vi "KalmanMain.vi"() -> ()   [LabVIEW 2017]
uses:
  <vilib>/Analysis/Matrix/Datatypes/RealMatrix.ctl
  4782e2db-7f08-4414-a468-fee53f76426c.vi
  <vilib>/Analysis/baseanly.llb/Real A x B.vi
  <vilib>/Analysis/Matrix/Numeric/Add/Add - RM,RM.vi
  <vilib>/Analysis/7linalg.llb/Create Special Real Matrix.vi
  <vilib>/Analysis/baseanly.llb/Real Inverse Matrix.vi
  <vilib>/Analysis/Matrix/Numeric/Subtract/Subtract - RM,RM.vi
  <vilib>/Analysis/NI_AALBase.lvlib
  <vilib>/Analysis/Matrix/NI_Matrix.lvlib
  <vilib>/Analysis/NI_AALPro.lvlib
panel:
  in  "delay":u32=500
  out "P 2":T1
  out "Xhat 2":T1
  in  "Xhat":T1=[[0.0], [0.0]]
  in  "Q":T1=[[1.0, 0.0], [0.0, 1.0]]
  in  "R":T1=[[1.0]]
  in  "H":T1=[[1.0, 0.0]]
  in  "A":T1=[[1.0, 1.0], [0.0, 1.0]]
  in  "P":T1=[[10.0, 0.0], [0.0, 10.0]]
  in  "Measurements":dbl[](array[numeric])=[1.0, 2.0, 3.0, 4.0]
  out "XY Graph":T2(graph)
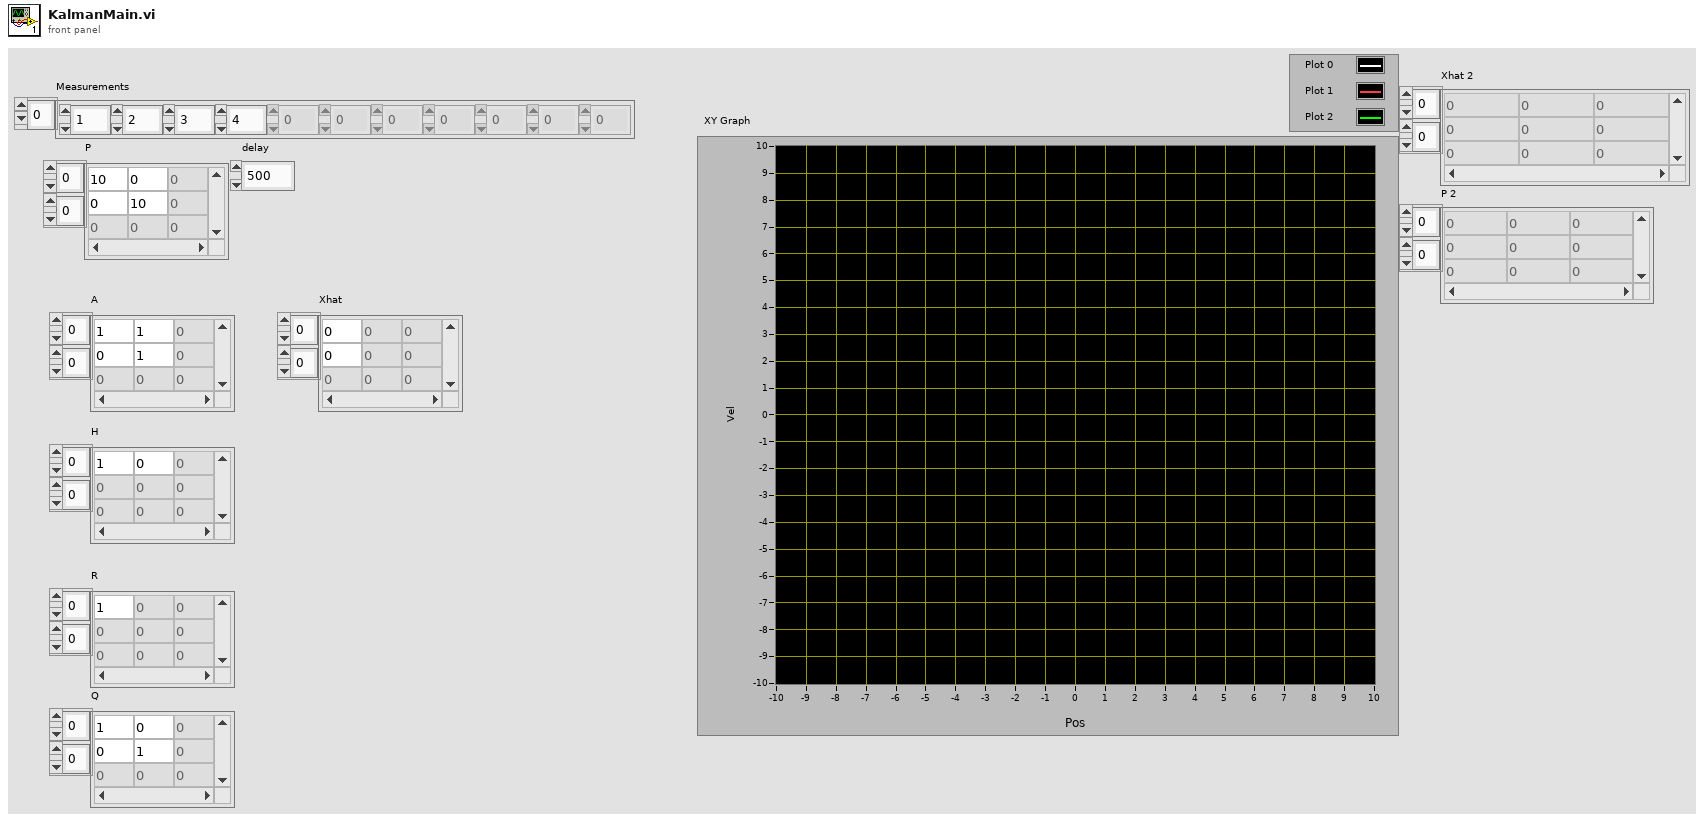
[diagram p1: front panel]
types:
  T1 = typedef "NI_Matrix.lvlib/RealMatrix.ctl" = dbl[][]
  T2 = cluster{"A x Vector":dbl[], "A x Vector":dbl[]}[]
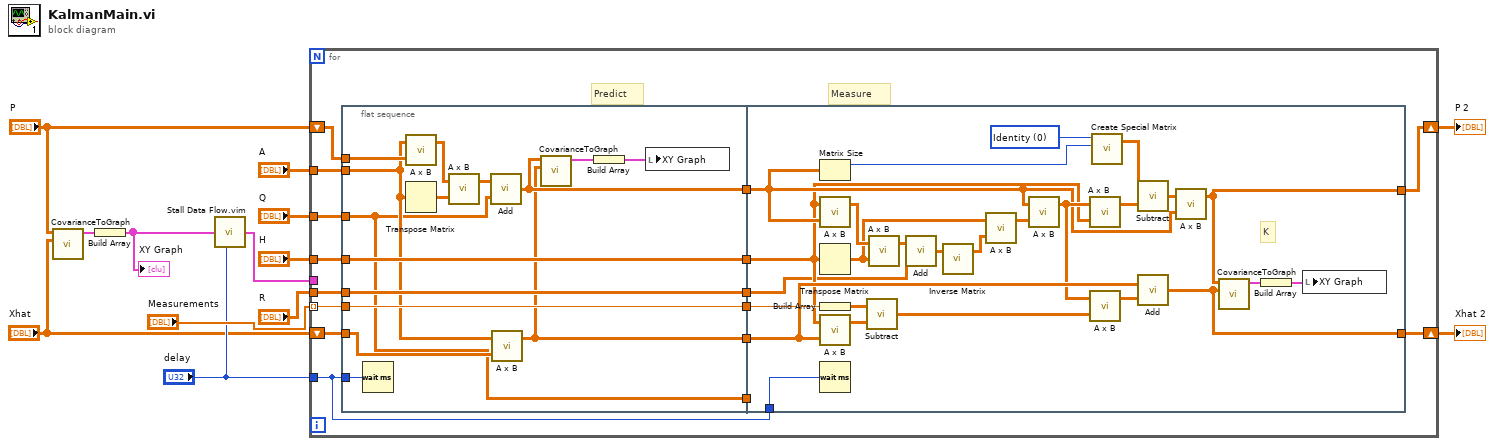
[diagram p0: block diagram]
diagram:
  n1 = call "CovarianceToGraph.vi"("Mu"="Xhat", "covariance matrix"="P") -> ("XY Graph"=w13:cluster{cdb[], cdb[]})  [unwired: 9 in]
  n2 = Build Array(w13) -> (w4:cluster{cdb[], cdb[]}[])
  "XY Graph" <- w4
  n3 = call "Stall Data Flow.vim"("value in"=w4, "milliseconds to wait"="delay") -> ("value out"=w3:cluster{cdb[], cdb[]}[])  [unwired: 1 out]
  n4 = for {
    tunnel: "Measurements" -> [w24] mode=indexing
    tunnel: "A" -> [w28]
    shift-right: [w19] -> w7
    shift-left: "Xhat" -> [w29]
    shift-right: [w18] -> w5
    shift-left: "P" -> [w27]
    tunnel: "H" -> [w26]
    tunnel: "R" -> [w25]
    tunnel: "Q" -> [w17]
    tunnel: w3 -> [_]
    tunnel: "delay" -> [w15]
    # "Predict"
    # "Measure"
    n5 = flat-sequence {
      tunnel: w24 -> [w42]
      tunnel: w25 -> [w43]
      tunnel: w26 -> [w44]
      tunnel: w27 -> [w40]
      tunnel: w28 -> [w39]
      tunnel: w29 -> [w41]
      tunnel: [w31] -> w23
      tunnel: [w44] -> w22
      tunnel: [w43] -> w21
      tunnel: [w42] -> w20
      tunnel: w17 -> [w30]
      tunnel: [w34] -> w16
      tunnel: w15 -> [w32]
      tunnel: [w30] -> w14
      tunnel: w23 -> [w63]
      tunnel: w22 -> [w46]
      tunnel: w21 -> [w45]
      tunnel: w20 -> [w47]
      tunnel: [w49] -> w19
      tunnel: [w48] -> w18
      tunnel: w16 -> [w54]
      tunnel: w15 -> [w52]
      tunnel: w14 -> [_]
      frame #0 {
        n6 = Wait (ms)(milliseconds to wait=w32) -> ()  [unwired: 1 out]
        n7 = call-poly <vilib>:"A x B.vi"("B"=w40, "A"=w39) -> ("A x B"=w38:T1)  [unwired: 1 out]
        n8 = Transpose Matrix(1:w39) -> (0:w37:T1)
        n9 = call-poly <vilib>:"A x B.vi"("B"=w37, "A"=w38) -> ("A x B"=w36:T1)  [unwired: 1 out]
        n10 = call-poly <vilib>:"Add.vi"("Real Matrix B"=w30, "Real Matrix A"=w36) -> ("A + B"=w34:T1)
        n11 = call-poly <vilib>:"A x B.vi"("B"=w41, "A"=w39) -> ("A x B"=w31:T1)  [unwired: 1 out]
        n12 = call "CovarianceToGraph.vi"("Mu"=w31, "covariance matrix"=w34) -> ("XY Graph"=w35:cluster{cdb[], cdb[]})  [unwired: 9 in]
        n13 = Build Array(w35) -> (w33:cluster{cdb[], cdb[]}[])
        n14 = local write "XY Graph"(w33) -> ()
      }
      frame #1 {
        w59 = 0 items=["Identity", "Diagonal", "Toeplitz", "Vandermonde", "Companion", "Hankel", "Hadamard", "Wilkinson", "Hilbert", "Inverse Hilbert", "Rosser", "Pascal"] ("matrix type")
        # "K"
        n15 = Matrix Size(0:w54) -> (1:w58:i32)  [unwired: 1 out]
        n16 = call-poly <vilib>:"A x B.vi"("B"=w54, "A"=w46) -> ("A x B"=w70:T1)  [unwired: 1 out]
        n17 = Transpose Matrix(1:w46) -> (0:w66:T1)
        n18 = Build Array(w47) -> (w64:T1)
        n19 = call-poly <vilib>:"A x B.vi"("B"=w63, "A"=w46) -> ("A x B"=w62:T1)  [unwired: 1 out]
        n20 = Wait (ms)(milliseconds to wait=w52) -> ()  [unwired: 1 out]
        n21 = call-poly <vilib>:"Subtract.vi"("Real Matrix B"=w62, "Real Matrix A"=w64) -> ("A - B"=w61:T1)
        n22 = call-poly <vilib>:"A x B.vi"("B"=w66, "A"=w70) -> ("A x B"=w69:T1)  [unwired: 1 out]
        n23 = call-poly <vilib>:"Add.vi"("Real Matrix B"=w45, "Real Matrix A"=w69) -> ("A + B"=w68:T1)
        n24 = call-poly <vilib>:"Inverse Matrix.vi"("Input Matrix"=w68) -> ("Inverse Matrix"=w67:T1)  [unwired: 1 in, 1 out]
        n25 = call-poly <vilib>:"A x B.vi"("B"=w67, "A"=w66) -> ("A x B"=w65:T1)  [unwired: 1 out]
        n26 = call-poly <vilib>:"A x B.vi"("B"=w65, "A"=w54) -> ("A x B"=w56:T1)  [unwired: 1 out]
        n27 = call-poly <vilib>:"A x B.vi"("B"=w46, "A"=w56) -> ("A x B"=w55:T1)  [unwired: 1 out]
        n28 = call-poly <vilib>:"A x B.vi"("B"=w61, "A"=w56) -> ("A x B"=w60:T1)  [unwired: 1 out]
        n29 = call-poly <vilib>:"Create Special Matrix.vi"("matrix type"=w59, "matrix size"=w58) -> ("Special Matrix"=w57:T1)  [unwired: 3 in, 1 out]
        n30 = call-poly <vilib>:"Subtract.vi"("Real Matrix B"=w55, "Real Matrix A"=w57) -> ("A - B"=w53:T1)
        n31 = call-poly <vilib>:"Add.vi"("Real Matrix B"=w60, "Real Matrix A"=w63) -> ("A + B"=w49:T1)
        n32 = call-poly <vilib>:"A x B.vi"("B"=w54, "A"=w53) -> ("A x B"=w48:T1)  [unwired: 1 out]
        n33 = call "CovarianceToGraph.vi"("Mu"=w49, "covariance matrix"=w48) -> ("XY Graph"=w50:cluster{cdb[], cdb[]})  [unwired: 9 in]
        n34 = Build Array(w50) -> (w51:cluster{cdb[], cdb[]}[])
        n35 = local write "XY Graph"(w51) -> ()
      }
    }
  }
  "Xhat 2" <- w7
  "P 2" <- w5
